vi "Read First Character.vi"(8 "Error In":errorcluster) -> (0 "Error Out":errorcluster)   [LabVIEW 2018, in "Tests.lvlib" / "Readers.lvlib" / "String.lvlib"]
uses:
  String.lvlib
  src/Mustache/Public/Readers/Public/String/String.lvclass
  <vilib>/addons/_JKI Toolkits/Caraya/classes/Test/Test.lvclass
  <vilib>/addons/_JKI Toolkits/Caraya/classes/Assert/Assert.lvclass
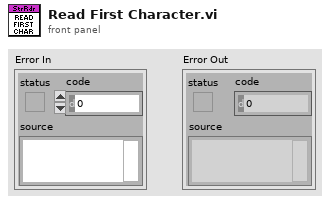
[diagram p1: front panel]
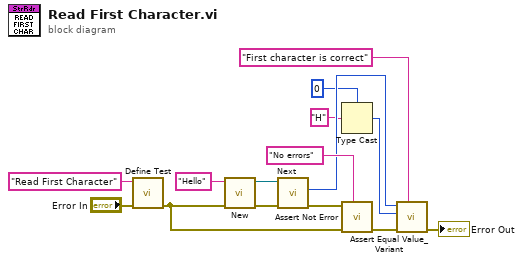
[diagram p0: block diagram]
diagram:
  n1 = call <vilib>:"Define Test.vi"("error in (no error)"="Error In", "Label (VI Title)"="Read First Character") -> ("error out"=w9:errorcluster)  [unwired: 9 in]
  n2 = call "New.vi"("Error In"=w9, "String"="Hello") -> ("Error Out"=w11:errorcluster, "String"=w12:refnum<class "String.lvclass">)  [unwired: 8 in]
  n3 = call-dynamic "Next.vi"("Error In"=w11, "Reader In"=w12) -> ("Error Out"=w10:errorcluster, "Character"=w5:u8)  [unwired: 6 in, 2 out]
  n4 = Type Cast(type=u8 0, x="H") -> (*(type *) &x=w1:u8)
  n5 = call <vilib>:"Assert Not Error.vi"("Label"="No errors", "error in (no error)"=w9, "Not Error?"=w10) -> ("error out"=w7:errorcluster)  [unwired: 8 in]
  n6 = call <vilib>:"Assert Equal Value_Variant.vi"("Label"="First character is correct", "error in (no error)"=w7, "Y"=w1, "X"=w5) -> ("error out"=→"Error Out":errorcluster)  [unwired: 7 in]
